vi "MB Serial Wait on Query.vi"(11 "VISA resource name":refnum<visa-resource-name>) -> ()   [LabVIEW 2011]
uses:
  MB RefCount Function.ctl
  MB Globals.vi
panel:
  in  "Serial Parameters":T1 {"Slave Address" format="%.0x"}
  in  "Timeout":u32=10000
  # "VI Name: MB Serial Wait on Query.vi\nPurpose: Serves a Modbus TCP query.\nReentrant VI called dynamically, so that multiple\nqueries can be served in parallel."
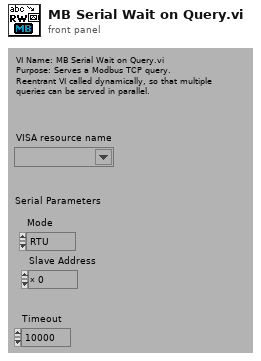
[diagram p1: front panel]
types:
  T1 = cluster{"Mode":enum16{"RTU", "ASCII"}, "Slave Address":u8}
  T2 = typedef "MB RefCount Function.ctl" = enum16{"Init", "Add", "Remove", "Is Running?"}
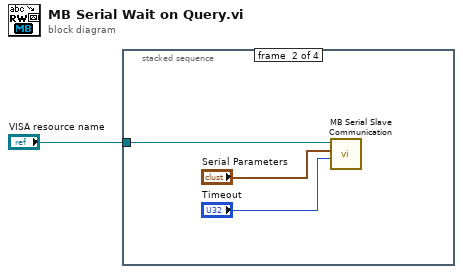
[diagram p0: block diagram]
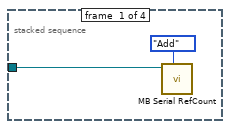
[diagram p2: hidden frame]
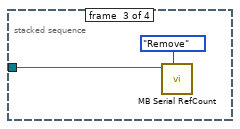
[diagram p3: hidden frame]
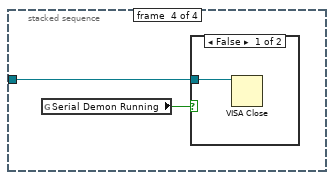
[diagram p4: hidden frame]
diagram:
  n1 = stacked-sequence {
    tunnel: "VISA resource name" -> [w2 w6 w7 w10]
    frame #0 {
      n2 = call "MB Serial RefCount.vi"("Function"=MB_RefCount_Function."Add", "VISA resource name"=w2) -> ()  [unwired: 10 out]
    }
    frame #1 {
      n3 = call "MB Serial Slave Communication.vi"("Timeout"="Timeout", "Serial Parameters"="Serial Parameters", "VISA resource name"=w6) -> ()  [unwired: 1 in, 8 out]
    }
    frame #2 {
      n4 = call "MB Serial RefCount.vi"("Function"=MB_RefCount_Function."Remove", "VISA resource name"=w7) -> ()  [unwired: 10 out]
    }
    frame #3 {
      n5 = global read "MB Globals.vi" "Serial Demon Running"() -> (w9:bool)
      n6 = case shown="False" w9 {
        tunnel: w10 -> [w11 _]
        frame False {
          n7 = VISA Close(VISA resource name=w11) -> ()  [unwired: 1 in, 1 out]
        }
        frame True {
        }
      }
    }
  }
